vi "Configure Output Phase.vi"(0 "VISA resource name":refnum<visa-resource-name>, 5 "Output Phase (0')":dbl format="%#.4g", 7 "Output Phase Mode (0: Fix)":u16(ring) items=["Fixed", "Step", "Pulse", "List"], 9 "Triggered Output Phase (0')":dbl format="%#.4g", 11 "error in (no error)":errorcluster) -> (4 "VISA resource name out":refnum<visa-resource-name>, 15 "error out":errorcluster)   [LabVIEW 2020, in "Agilent 681x Series.lvlib"]
doc: "Configures the phase settings of the output voltage waveform."
uses:
  <instrlib>/Agilent 681x Series/Agilent 681x Series.lvlib
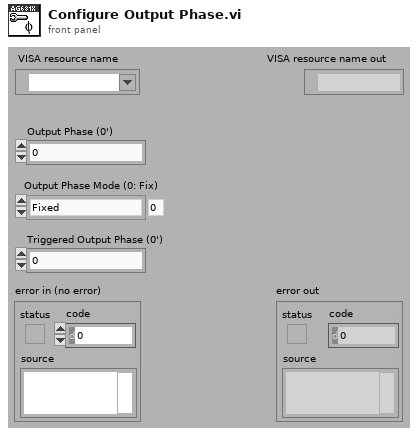
[diagram p1: front panel]
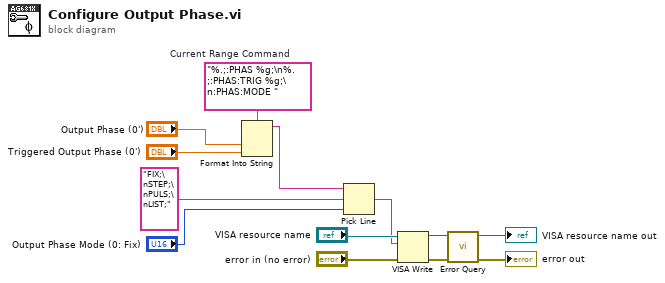
[diagram p0: block diagram]
diagram:
  w9 = "%.;:PHAS %g;\n%.;:PHAS:TRIG %g;\n:PHAS:MODE "  # Current Range Command
  n1 = Format Into String(format string=w9, "Output Phase (0')", "Triggered Output Phase (0')") -> (resulting string=w5:string)  [unwired: 2 in, 1 out]
  n2 = Pick Line(string ("")=w5, multi-line string="FIX;\nSTEP;\nPULS;\nLIST;", line index="Output Phase Mode (0: Fix)") -> (output string=w2:string)
  n3 = VISA Write(VISA resource name="VISA resource name", write buffer=w2, error in (no error)="error in (no error)") -> (VISA resource name out=w11:refnum<visa-resource-name>, error out=w10:errorcluster)  [unwired: 1 out]
  n4 = call <instrlib>:"Error Query.vi"("error in (no error)"=w10, "VISA resource name"=w11) -> ("error out"=→"error out":errorcluster, "VISA resource name out"=→"VISA resource name out":refnum<visa-resource-name>)  [unwired: 6 in, 2 out]
